vi "DETT Record Run Debug Info.vi"(0 "Exec.State":T1(ring), 1 "Button Text":string, 2 "Exec.IsReentrant":bool, 3 "Path":path) -> ()   [LabVIEW 2011, in "Generic Plugin.lvclass"]
uses:
  Generic Plugin.lvclass
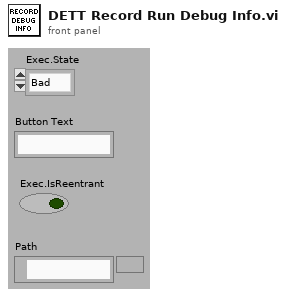
[diagram p1: front panel]
types:
  T1 = enum32{"Bad", "Idle", "Run top level", "Running"}
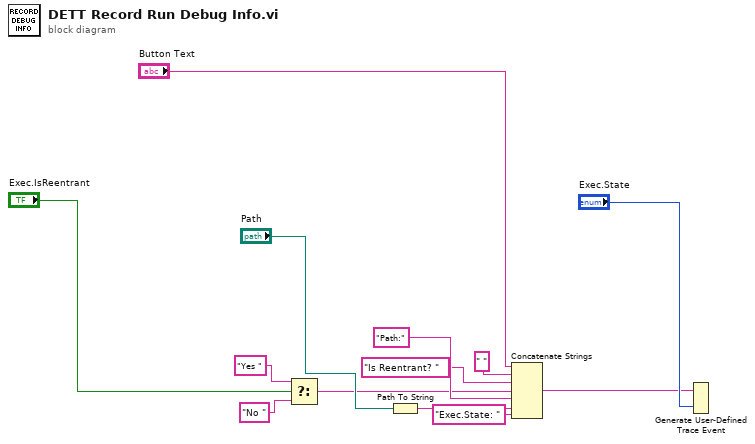
[diagram p0: block diagram]
diagram:
  n1 = Select(t="Yes " ("string"), s="Exec.IsReentrant", f="No " ("string")) -> (s? t:f=w5:string)
  n2 = Path To String(path="Path") -> (string=w9:string)
  n3 = Concatenate Strings("Button Text", " " ("string"), "Is Reentrant? " ("string"), w5, "Path:" ("string"), w9, "Exec.State: " ("string")) -> (w11:string)
  n4 = Generate User-Defined Trace Event(1:"Exec.State", 2:w11) -> ()
